vi "Dodawanie położeń robota do mapy.vi"(7 "Poł. startowe\n piksele":cluster{"X":i32, "Y":i32}, 8 "error in (no error)":errorcluster, 9 "Dł. piksela [m]":dbl, 10 "Mapa terenu":picture, 11 "Dane z położenia":refnum<queue>) -> (0 "error out":errorcluster, 1 "Odległość robota od startu [m]":cluster{"X [m]":dbl, "Y [m]":dbl}, 2 "Mapa z wprowadzonym punktem":picture)   [LabVIEW 2012, in "Biblioteka moduł map v3.lvlib" / "Pomocnicze.lvlib"]
uses:
  Pomocnicze.lvlib
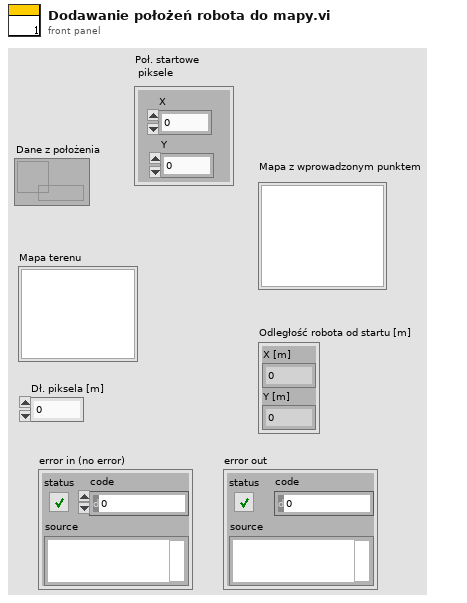
[diagram p1: front panel]
types:
  T1 = cluster{"Width":u16, "Style":enum32{"Solid", "Dash", "Dot", "DashDot", "DashDotDot"}}
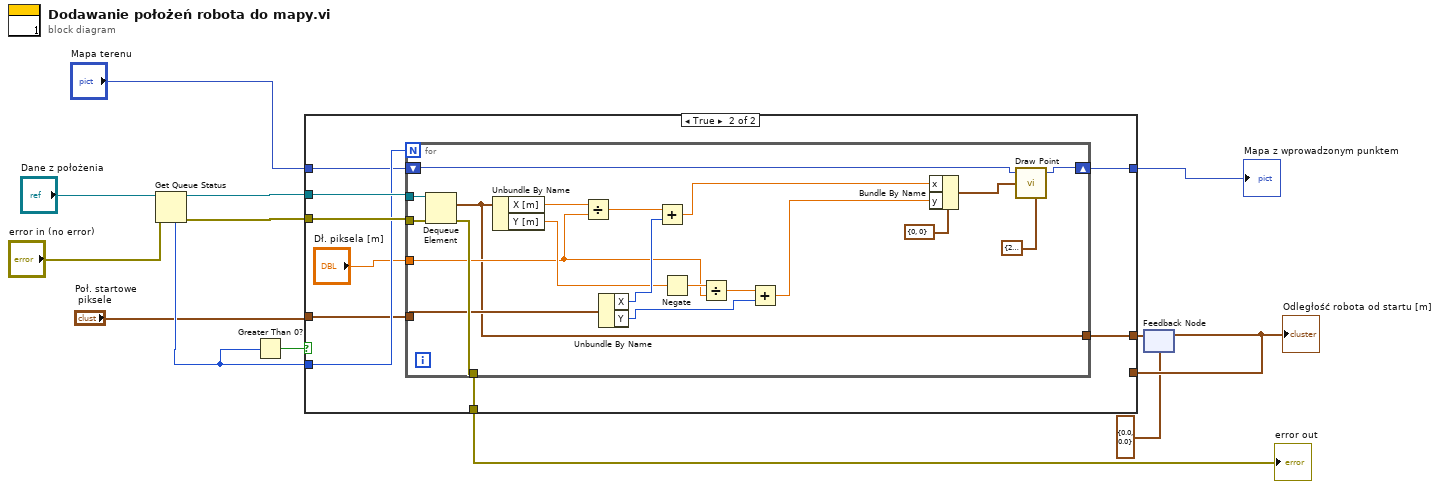
[diagram p0: block diagram]
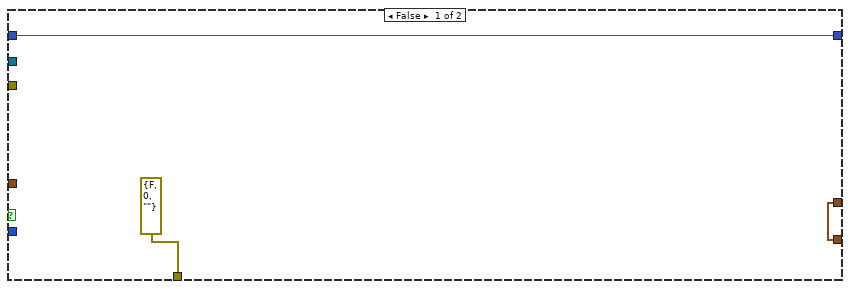
[diagram p2: hidden frame]
diagram:
  n1 = Get Queue Status(queue="Dane z położenia", error in (no error)="error in (no error)") -> (queue out=w10:refnum<queue>, error out=w11:errorcluster, # elements in queue=w13:i32)  [unwired: 1 in, 5 out]
  n2 = Greater Than 0?(x=w13) -> (x > 0?=w3:bool)
  n3 = feedback #1(cluster{"X [m]":dbl, "Y [m]":dbl} {"X [m]"=0.0, "Y [m]"=0.0}) -> (w4:cluster{"X [m]":dbl, "Y [m]":dbl})
  "Odległość robota od startu [m]" <- w4
  n4 = case shown="True" w3 {
    tunnel: w10 -> [_ w25]
    tunnel: w11 -> [_ w24]
    tunnel: [errorcluster {"status"=FALSE, "code"=0, "source"=""} ("error out") w23] -> w12
    tunnel: w13 -> [_ w22]
    tunnel: [w15 w21] -> w7
    tunnel: "Mapa terenu" -> [w15 w20]
    tunnel: "Poł. startowe\n piksele" -> [_ w19]
    tunnel: [w14 w17] -> w2
    tunnel: w4 -> [w14 _]
    frame False {
    }
    frame True {
      n5 = for {
        N: w22 -> [_]
        tunnel: w25 -> [w45]
        tunnel: w24 -> [w44]
        tunnel: [w43] -> w23
        shift-right: [w30] -> w21
        shift-left: w20 -> [w29]
        tunnel: w19 -> [w33]
        tunnel: "Dł. piksela [m]" -> [w32]
        tunnel: [w31] -> w17
        n6 = Dequeue Element(queue=w45, error in (no error)=w44) -> (element=w31:cluster{"X [m]":dbl, "Y [m]":dbl}, error out=w43:errorcluster)  [unwired: 1 in, 2 out]
        n7 = Unbundle By Name(w31) -> ("X [m]"=w35:dbl, "Y [m]"=w34:dbl)
        n8 = Divide(x=w35, y=w32) -> (x/y=w39:dbl)
        n9 = Unbundle By Name(w33) -> ("X"=w41:i32, "Y"=w42:i32)
        n10 = Add(x=w39, y=w41) -> (x+y=w40:dbl)
        n11 = Negate(x=w34) -> (-x=w36:dbl)
        n12 = Divide(x=w36, y=w32) -> (x/y=w37:dbl)
        n13 = Add(x=w37, y=w42) -> (x+y=w38:dbl)
        n14 = Bundle By Name(cluster=cluster{"x":i16, "y":i16} {"x"=0, "y"=0} ("point(x,y)"), "x"=w40, "y"=w38) -> (w26:cluster{"x":i16, "y":i16})
        n15 = call <vilib>:"Draw Point.vi"("picture"=w29, "point(x,y)"=w26, "pen"=T1 {"Width"=2, "Style"=enum."Solid"}) -> ("new picture"=w30:picture)  [unwired: 6 in]
      }
    }
  }
  "error out" <- w12
  "Mapa z wprowadzonym punktem" <- w7
  n16 = feedback-in #1(w2) -> ()
